vi "Control Sys Motor Control.vi"   [LabVIEW 2015]
uses:
  Localization/Right Variables.vi
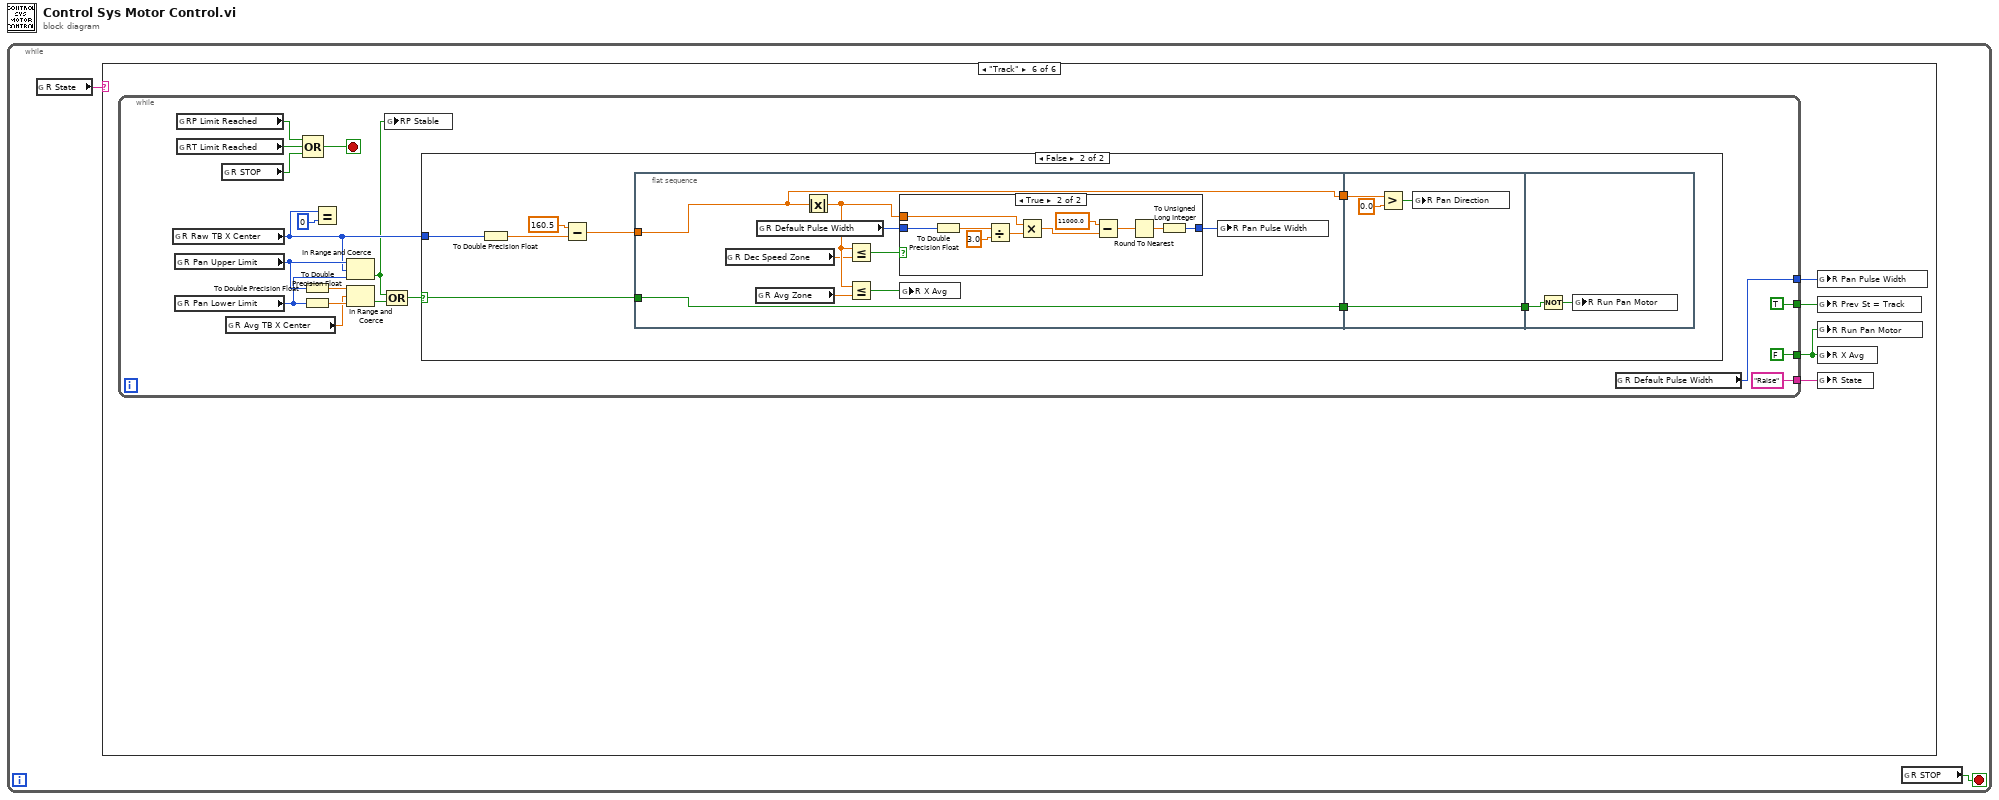
[diagram p0: block diagram]
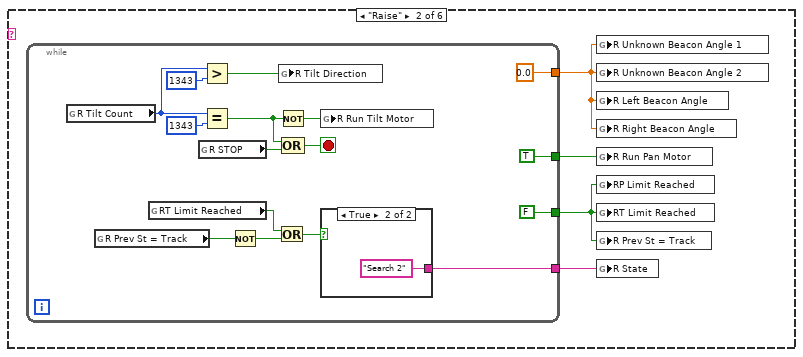
[diagram p3: hidden frame]
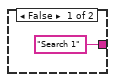
[diagram p4: hidden frame]
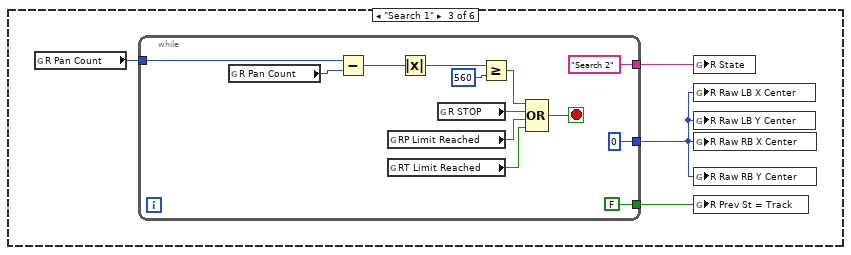
[diagram p5: hidden frame]
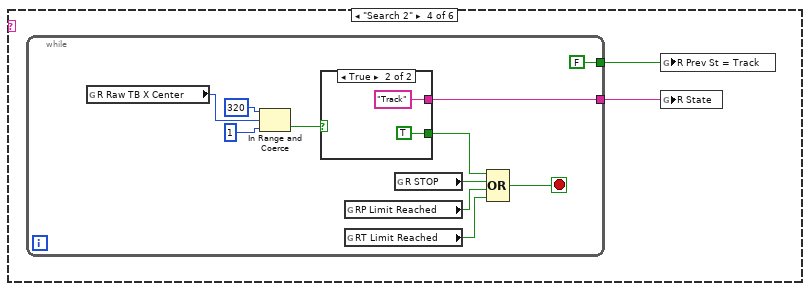
[diagram p6: hidden frame]
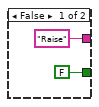
[diagram p7: hidden frame]
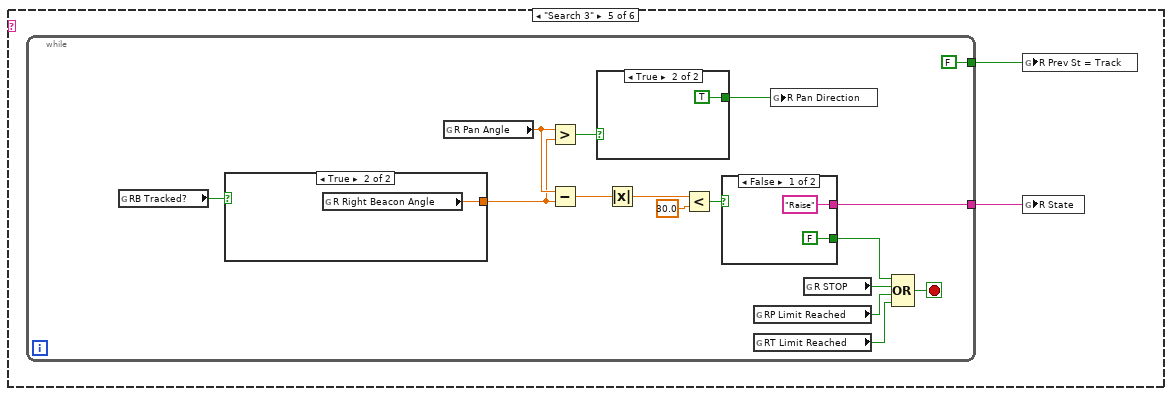
[diagram p8: hidden frame]
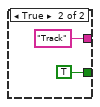
[diagram p9: hidden frame]
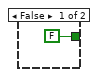
[diagram p10: hidden frame]
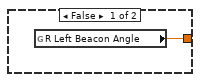
[diagram p11: hidden frame]
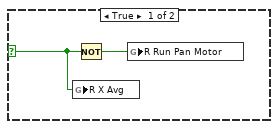
[diagram p12: hidden frame]
diagram:
  n1 = while {
    stop <- w1 stop-if-true
    n2 = global read "Right Variables.vi" "R State"() -> (w2:string)
    n3 = case shown="\"Track\"" w2 {
      frame "Null", Default {
      }
      frame "Raise" {
        n4 = while {
          tunnel: [w21] -> w6
          tunnel: [FALSE] -> w3
          tunnel: [TRUE ("L Run Pan Motor")] -> w5
          tunnel: [0.0] -> w4
          stop <- w22 stop-if-true
          n5 = global read "Right Variables.vi" "R Tilt Count"() -> (w17:i32)
          n6 = global read "Right Variables.vi" "R Prev St = Track"() -> (w10:bool)
          n7 = global read "Right Variables.vi" "RT Limit Reached"() -> (w8:bool)
          n8 = global read "Right Variables.vi" "R STOP"() -> (w14:bool)
          n9 = Greater?(x=w17, y=1343) -> (0:w15:bool)
          n10 = Equal?(x=w17, y=1343) -> (x = y?=w18:bool)
          n11 = Not(x=w10) -> (.not. x?=w9:bool)
          n12 = Or(x=w8, y=w9) -> (x .or. y?=w7:bool)
          n13 = Not(x=w18) -> (.not. x?=w16:bool)
          n14 = global write "Right Variables.vi" "R Tilt Direction"(w15) -> ()
          n15 = Compound Arithmetic op=OR(w18, w14) -> (w22:bool)
          n16 = global write "Right Variables.vi" "R Run Tilt Motor"(w16) -> ()
          n17 = case shown="True" w7 {
            tunnel: ["Search 1" ("L State") "Search 2" ("L State")] -> w21
            frame False {
            }
            frame True {
            }
          }
        }
        n18 = global write "Right Variables.vi" "R Unknown Beacon Angle 1"(w4) -> ()
        n19 = global write "Right Variables.vi" "R Unknown Beacon Angle 2"(w4) -> ()
        n20 = global write "Right Variables.vi" "R Left Beacon Angle"(w4) -> ()
        n21 = global write "Right Variables.vi" "R Right Beacon Angle"(w4) -> ()
        n22 = global write "Right Variables.vi" "R Run Pan Motor"(w5) -> ()
        n23 = global write "Right Variables.vi" "RP Limit Reached"(w3) -> ()
        n24 = global write "Right Variables.vi" "RT Limit Reached"(w3) -> ()
        n25 = global write "Right Variables.vi" "R Prev St = Track"(w3) -> ()
        n26 = global write "Right Variables.vi" "R State"(w6) -> ()
      }
      frame "Search 1" {
        n27 = global read "Right Variables.vi" "R Pan Count"() -> (w28:i32)
        n28 = while {
          tunnel: ["Search 2"] -> w27
          tunnel: w28 -> [w37]
          tunnel: [u16 0] -> w26
          tunnel: [FALSE] -> w25
          stop <- w41 stop-if-true
          n29 = global read "Right Variables.vi" "R Pan Count"() -> (w34:i32)
          n30 = Subtract(x=w37, y=w34) -> (x-y=w36:i32)
          n31 = global read "Right Variables.vi" "RP Limit Reached"() -> (w31:bool)
          n32 = global read "Right Variables.vi" "RT Limit Reached"() -> (w30:bool)
          n33 = Absolute Value(x=w36) -> (abs(x)=w35:i32)
          n34 = global read "Right Variables.vi" "R STOP"() -> (w33:bool)
          n35 = Greater Or Equal?(x=w35, y=560) -> (x >= y?=w38:bool)
          n36 = Compound Arithmetic op=OR(w38, w33, w31, w30) -> (w41:bool)
        }
        n37 = global write "Right Variables.vi" "R State"(w27) -> ()
        n38 = global write "Right Variables.vi" "R Raw LB X Center"(w26) -> ()
        n39 = global write "Right Variables.vi" "R Raw LB Y Center"(w26) -> ()
        n40 = global write "Right Variables.vi" "R Raw RB X Center"(w26) -> ()
        n41 = global write "Right Variables.vi" "R Raw RB Y Center"(w26) -> ()
        n42 = global write "Right Variables.vi" "R Prev St = Track"(w25) -> ()
      }
      frame "Search 2" {
        n43 = while {
          tunnel: [w48] -> w43
          tunnel: [FALSE] -> w42
          stop <- w52 stop-if-true
          n44 = global read "Right Variables.vi" "R Raw TB X Center"() -> (w49:u16)
          n45 = In Range and Coerce(upper limit=u16 320, x=w49, lower limit=u16 1) -> (In Range?=w50:bool)  [unwired: 1 out]
          n46 = case shown="True" w50 {
            tunnel: ["Raise" "Track"] -> w48
            tunnel: [FALSE TRUE] -> w47
            frame False {
            }
            frame True {
            }
          }
          n47 = global read "Right Variables.vi" "RP Limit Reached"() -> (w46:bool)
          n48 = global read "Right Variables.vi" "RT Limit Reached"() -> (w45:bool)
          n49 = global read "Right Variables.vi" "R STOP"() -> (w51:bool)
          n50 = Compound Arithmetic op=OR(w47, w51, w46, w45) -> (w52:bool)
        }
        n51 = global write "Right Variables.vi" "R Prev St = Track"(w42) -> ()
        n52 = global write "Right Variables.vi" "R State"(w43) -> ()
      }
      frame "Search 3" {
        n53 = while {
          tunnel: [w62] -> w60
          tunnel: [FALSE] -> w59
          stop <- w67 stop-if-true
          n54 = global read "Right Variables.vi" "RB Tracked?"() -> (w76:bool)
          n55 = case shown="True" w76 {
            tunnel: [w83 w84] -> w72
            frame False {
              n56 = global read "Right Variables.vi" "R Left Beacon Angle"() -> (w83:dbl)
            }
            frame True {
              n57 = global read "Right Variables.vi" "R Right Beacon Angle"() -> (w84:dbl)
            }
          }
          n58 = global read "Right Variables.vi" "R Pan Angle"() -> (w73:dbl)
          n59 = Greater?(x=w73, y=w72) -> (0:w75:bool)
          n60 = Subtract(x=w73, y=w72) -> (x-y=w64:dbl)
          n61 = case shown="True" w75 {
            tunnel: [FALSE TRUE] -> w74
            frame False {
            }
            frame True {
            }
          }
          n62 = Absolute Value(x=w64) -> (abs(x)=w63:dbl)
          n63 = Less?(x=w63, y=30.0) -> (x < y?=w70:bool)
          n64 = case shown="False" w70 {
            tunnel: ["Raise" "Track"] -> w62
            tunnel: [FALSE TRUE] -> w69
            frame False {
            }
            frame True {
            }
          }
          n65 = global read "Right Variables.vi" "RP Limit Reached"() -> (w66:bool)
          n66 = global read "Right Variables.vi" "RT Limit Reached"() -> (w65:bool)
          n67 = global write "Right Variables.vi" "R Pan Direction"(w74) -> ()
          n68 = global read "Right Variables.vi" "R STOP"() -> (w68:bool)
          n69 = Compound Arithmetic op=OR(w69, w68, w66, w65) -> (w67:bool)
        }
        n70 = global write "Right Variables.vi" "R Prev St = Track"(w59) -> ()
        n71 = global write "Right Variables.vi" "R State"(w60) -> ()
      }
      frame "Track" {
        n72 = while {
          tunnel: ["Raise"] -> w88
          tunnel: [FALSE] -> w87
          tunnel: [TRUE] -> w86
          tunnel: [w89] -> w85
          stop <- w106 stop-if-true
          n73 = global read "Right Variables.vi" "R Raw TB X Center"() -> (w94:u16)
          n74 = global read "Right Variables.vi" "R Pan Upper Limit"() -> (w101:u16)
          n75 = global read "Right Variables.vi" "R Pan Lower Limit"() -> (w100:u16)
          n76 = global read "Right Variables.vi" "RP Limit Reached"() -> (w96:bool)
          n77 = global read "Right Variables.vi" "RT Limit Reached"() -> (w98:bool)
          n78 = global read "Right Variables.vi" "R STOP"() -> (w97:bool)
          n79 = global read "Right Variables.vi" "R Avg TB X Center"() -> (w99:dbl)
          n80 = Compound Arithmetic op=OR(w96, w98, w97) -> (w106:bool)
          n81 = To Double Precision Float(number=w101) -> (double precision float=w104:dbl)
          n82 = To Double Precision Float(number=w100) -> (double precision float=w103:dbl)
          n83 = Equal?(x=w94, y=u16 0) -> ()  [unwired: 1 out]
          n84 = In Range and Coerce(upper limit=w101, x=w94, lower limit=w100) -> (In Range?=w92:bool)  [unwired: 1 out]
          n85 = In Range and Coerce(upper limit=w104, x=w99, lower limit=w103) -> (In Range?=w102:bool)  [unwired: 1 out]
          n86 = global write "Right Variables.vi" "RP Stable"(w92) -> ()
          n87 = Compound Arithmetic op=OR(w92, w102) -> (w91:bool)
          n88 = case shown="False" w91 {
            selector: w91 -> [w108 w109]
            tunnel: w94 -> [_ w116]
            frame True {
              n89 = global write "Right Variables.vi" "R X Avg"(w108) -> ()
              n90 = Not(x=w108) -> (.not. x?=w107:bool)
              n91 = global write "Right Variables.vi" "R Run Pan Motor"(w107) -> ()
            }
            frame False {
              n92 = To Double Precision Float(number=w116) -> (double precision float=w114:dbl)
              n93 = Subtract(x=160.5, y=w114) -> (x-y=w113:dbl)
              n94 = flat-sequence {
                tunnel: w113 -> [w118]
                tunnel: [w118] -> w112
                tunnel: [w117] -> w110
                tunnel: w109 -> [w117]
                tunnel: w112 -> [w138]
                tunnel: [w137] -> w111
                tunnel: w110 -> [w137]
                tunnel: w111 -> [w141]
                frame #0 {
                  n95 = global read "Right Variables.vi" "R Dec Speed Zone"() -> (w122:dbl)
                  n96 = global read "Right Variables.vi" "R Avg Zone"() -> (w123:dbl)
                  n97 = global read "Right Variables.vi" "R Default Pulse Width"() -> (w121:u32)
                  n98 = Absolute Value(x=w118) -> (abs(x)=w124:dbl)
                  n99 = Less Or Equal?(x=w124, y=w122) -> (x <= y?=w125:bool)
                  n100 = Less Or Equal?(x=w124, y=w123) -> (x <= y?=w120:bool)
                  n101 = case shown="True" w125 {
                    tunnel: w121 -> [w126 w136]
                    tunnel: [w126 w129] -> w119
                    tunnel: w124 -> [_ w127]
                    frame False {
                    }
                    frame True {
                      n102 = To Double Precision Float(number=w136) -> (double precision float=w128:dbl)
                      n103 = Divide(x=w128, y=3.0) -> (x/y=w133:dbl)
                      n104 = Multiply(x=w127, y=w133) -> (x*y=w132:dbl)
                      n105 = Subtract(x=11000.0, y=w132) -> (x-y=w131:dbl)
                      n106 = Round To Nearest(number=w131) -> (nearest integer value=w130:dbl)
                      n107 = To Unsigned Long Integer(number=w130) -> (unsigned 32bit integer=w129:u32)
                    }
                  }
                  n108 = global write "Right Variables.vi" "R X Avg"(w120) -> ()
                  n109 = global write "Right Variables.vi" "R Pan Pulse Width"(w119) -> ()
                }
                frame #1 {
                  n110 = Greater?(x=w138, y=0.0) -> (0:w140:bool)
                  n111 = global write "Right Variables.vi" "R Pan Direction"(w140) -> ()
                }
                frame #2 {
                  n112 = Not(x=w141) -> (.not. x?=w142:bool)
                  n113 = global write "Right Variables.vi" "R Run Pan Motor"(w142) -> ()
                }
              }
            }
          }
          n114 = global read "Right Variables.vi" "R Default Pulse Width"() -> (w89:u32)
        }
        n115 = global write "Right Variables.vi" "R Pan Pulse Width"(w85) -> ()
        n116 = global write "Right Variables.vi" "R Prev St = Track"(w86) -> ()
        n117 = global write "Right Variables.vi" "R Run Pan Motor"(w87) -> ()
        n118 = global write "Right Variables.vi" "R X Avg"(w87) -> ()
        n119 = global write "Right Variables.vi" "R State"(w88) -> ()
      }
    }
    n120 = global read "Right Variables.vi" "R STOP"() -> (w1:bool)
  }
